vi "map_tool_to_subsystem.vi"(7 "Tool Assignments":T1, 11 "Tool #":string) -> (3 "Subsystem out":string)   [LabVIEW 2017, in "labview-standard-library.lvlib" / "automode-scripting.lvlib"]
uses:
  automode-scripting.lvlib
  type-defs/tool-assignments.ctl
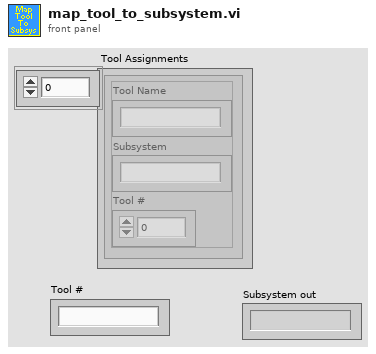
[diagram p1: front panel]
types:
  T1 = typedef "tool-assignments.ctl" = cluster{"Tool Name":string, "Subsystem":string, "Tool #":i32}[]
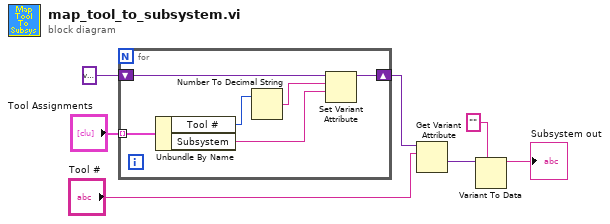
[diagram p0: block diagram]
diagram:
  n1 = for {
    shift-right: [w13] -> w4
    shift-left: variant -> [w12]
    tunnel: "Tool Assignments" -> [w11] mode=indexing
    n2 = Unbundle By Name(w11) -> ("Tool #"=w9:i32, "Subsystem"=w10:string)
    n3 = Number To Decimal String(number=w9) -> (decimal integer string=w8:string)  [unwired: 1 in]
    n4 = Set Variant Attribute(Variant=w12, name=w8, value=w10) -> (Variant out=w13:variant)  [unwired: 1 in, 2 out]
  }
  n5 = Get Variant Attribute(Variant=w4, name="Tool #") -> (value=w5:variant)  [unwired: 2 in, 3 out]
  n6 = Variant To Data(type="", Variant=w5) -> (data=→"Subsystem out":string)  [unwired: 1 in, 1 out]
